vi "Motion Status Reader.vi"(8 "error in (no error)":errorcluster, 11 "Control":refnum<notifier>) -> ()   [LabVIEW 2015, in "Tool Module.lvlib"]
uses:
  Tool Module.lvlib
  Tool Interface/_Host - HS Data Stream State Enum Typedef.ctl
  _Motion Status Reader SM enum--typedef.ctl
  Tool Typedefs/_Motion STATUS Cluster--typedef.ctl
  Tool Interface/GLOB - Configuration Options.vi
  Support/ToolModGLOB.vi
  Tool Interface/Tool Interface.lvlib
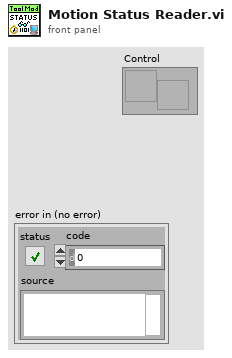
[diagram p1: front panel]
types:
  T1 = typedef "Tool Module.lvlib/_Motion Status Reader SM enum--typedef.ctl" = enum16{"Not Connected", "Connect", "Idle", "Receive Data", "Disconnect"}
  T2 = typedef "Tool Interface.lvlib/_Host - HS Data Stream State Enum Typedef.ctl" = enum16{"Idle", "Connect", "Receive Data", "Close Connection"}
  T3 = typedef "_Motion STATUS Cluster--typedef.ctl" = cluster{"Encoder":i32, "STATUS":u16, "MC SM State":u16, "M_Ctrl":u16}
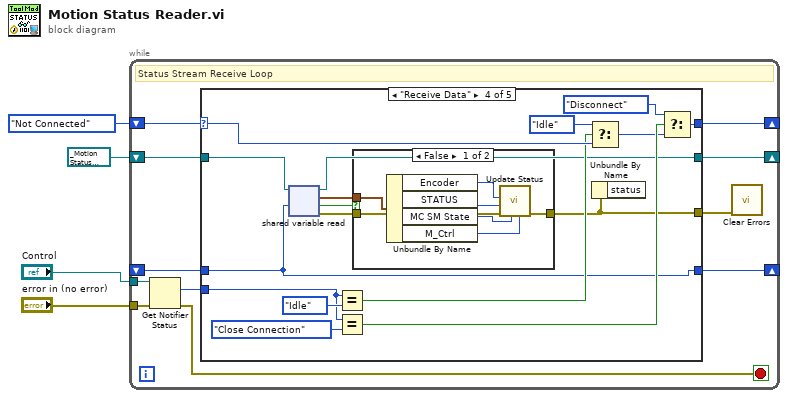
[diagram p0: block diagram]
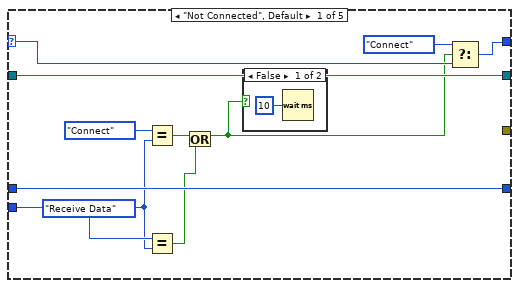
[diagram p2: hidden frame]
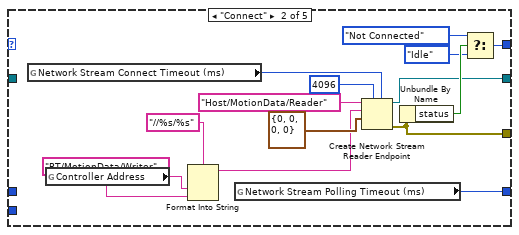
[diagram p4: hidden frame]
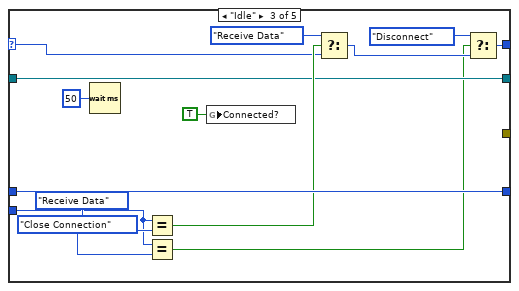
[diagram p5: hidden frame]
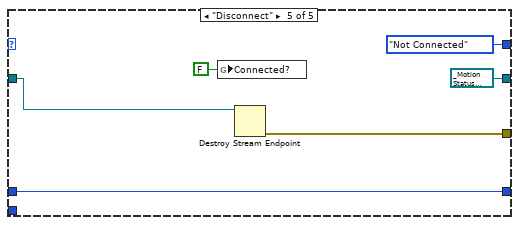
[diagram p7: hidden frame]
diagram:
  n1 = while {
    shift-right: [w14] -> _
    shift-left: _ -> [w13]
    shift-right: [w12] -> _
    shift-left: refnum<k21> refnum ("reader endpoint") -> [w7]
    tunnel: "Control" -> [w11]
    shift-right: [w9] -> _
    shift-left: _Motion_Status_Reader_SM_enum--typedef."Not Connected" ("_Motion Status Reader SM Enum--typedef") -> [w15]
    tunnel: "error in (no error)" -> [w6]
    stop <- w5 stop-if-true
    # "Status Stream Receive Loop"
    n2 = Get Notifier Status(notifier=w11, error in (no error)=w6) -> (current notification=w10:T2, error out=w5:errorcluster)  [unwired: 3 out]
    n3 = case shown="\"Receive Data\"" w15 {
      selector: w15 -> [w26 _ w53 w72 _]
      tunnel: [w23 w34 w55 w61 w84] -> w14
      tunnel: w13 -> [w23 _ w55 w61 w84]
      tunnel: [w22 w28 w51 w62 refnum<k21> refnum ("reader endpoint")] -> w12
      tunnel: w10 -> [w18 _ w44 w68 _]
      tunnel: [w25 w32 w50 w70 _Motion_Status_Reader_SM_enum--typedef."Not Connected" ("_Motion Status Reader SM Enum--typedef")] -> w9
      tunnel: [_ w33 _ w57 w85] -> w8
      tunnel: w7 -> [w22 _ w51 w63 w87]
      frame "Not Connected", Default {
        n4 = Equal?(x=_Host_-_HS_Data_Stream_State_Enum_Typedef."Connect", y=w18) -> (x = y?=w20:bool)
        n5 = Equal?(x=_Host_-_HS_Data_Stream_State_Enum_Typedef."Receive Data", y=w18) -> (x = y?=w16:bool)
        n6 = Or(x=w20, y=w16) -> (x .or. y?=w17:bool)
        n7 = case shown="False" w17 {
          frame False {
            n8 = Wait (ms)(milliseconds to wait=u32 10) -> ()  [unwired: 1 out]
          }
          frame True {
          }
        }
        n9 = Select(t=_Motion_Status_Reader_SM_enum--typedef."Connect", s=w17, f=w26) -> (s? t:f=w25:T1)
      }
      frame "Connect" {
        n10 = global read "GLOB - Configuration Options.vi" "Network Stream Connect Timeout (ms)"() -> (w39:i32)
        n11 = global read "GLOB - Configuration Options.vi" "Controller Address"() -> (w42:string)
        n12 = Format Into String(format string="//%s/%s", w42, "RT/MotionData/Writer" ("input 2")) -> (resulting string=w38:string)  [unwired: 2 in, 1 out]
        n13 = global read "GLOB - Configuration Options.vi" "Network Stream Polling Timeout (ms)"() -> (w34:i32)
        n14 = Create Network Stream Reader Endpoint(5:w39, 7:4096 ("reader buffer size"), 9:T3 {"Encoder"=0, "STATUS"=0, "MC SM State"=0, "M_Ctrl"=0} ("_Motion Status Cluster--typedef"), 10:w38, 11:"Host/MotionData/Reader" ("reader name")) -> (0:w33:errorcluster, 3:w28:refnum<k21>)  [unwired: 2 in]
        n15 = Unbundle By Name(w33) -> ("status"=w31:bool)
        n16 = Select(t=_Motion_Status_Reader_SM_enum--typedef."Not Connected", s=w31, f=_Motion_Status_Reader_SM_enum--typedef."Idle") -> (s? t:f=w32:T1)
      }
      frame "Idle" {
        n17 = Wait (ms)(milliseconds to wait=u32 50) -> ()  [unwired: 1 out]
        n18 = Equal?(x=w44, y=_Host_-_HS_Data_Stream_State_Enum_Typedef."Receive Data" ("x")) -> (x = y?=w54:bool)
        n19 = Equal?(x=w44, y=_Host_-_HS_Data_Stream_State_Enum_Typedef."Close Connection" ("x")) -> (x = y?=w47:bool)
        n20 = global write "ToolModGLOB.vi" "Connected?"(TRUE ("Connected?")) -> ()
        n21 = Select(t=_Motion_Status_Reader_SM_enum--typedef."Receive Data", s=w54, f=w53) -> (s? t:f=w49:T1)
        n22 = Select(t=_Motion_Status_Reader_SM_enum--typedef."Disconnect", s=w47, f=w49) -> (s? t:f=w50:T1)
      }
      frame "Receive Data" {
        n23 = shared-variable-read(w63, w61) -> (w62:refnum<k21>, w60:errorcluster, w58:bool, w59:T3)  [unwired: 1 in]
        n24 = Equal?(x=w68, y=_Host_-_HS_Data_Stream_State_Enum_Typedef."Idle" ("x")) -> (x = y?=w69:bool)
        n25 = Equal?(x=w68, y=_Host_-_HS_Data_Stream_State_Enum_Typedef."Close Connection") -> (x = y?=w66:bool)
        n26 = case shown="False" w58 {
          tunnel: w60 -> [w80 w81]
          tunnel: [w76 w81] -> w57
          tunnel: w59 -> [w79 _]
          frame False {
            n27 = Unbundle By Name(w79) -> ("Encoder"=w78:i32, "STATUS"=w77:u16, "MC SM State"=w75:u16, "M_Ctrl"=w74:u16)
            n28 = call "Update Status.vi"("M_Ctrl"=w74, "MC SM State"=w75, "error in (no error)"=w80, "STATUS"=w77, "Encoder"=w78) -> ("error out"=w76:errorcluster)  [unwired: 6 in]
          }
          frame True {
          }
        }
        n29 = Select(t=_Motion_Status_Reader_SM_enum--typedef."Idle", s=w69, f=w72) -> (s? t:f=w65:T1)
        n30 = Unbundle By Name(w57) -> ()  [unwired: 1 out]
        n31 = Select(t=_Motion_Status_Reader_SM_enum--typedef."Disconnect", s=w66, f=w65) -> (s? t:f=w70:T1)
      }
      frame "Disconnect" {
        n32 = global write "ToolModGLOB.vi" "Connected?"(FALSE ("Connected?")) -> ()
        n33 = Destroy Stream Endpoint(11:w87) -> (0:w85:errorcluster)  [unwired: 1 in]
      }
    }
    n34 = call <vilib>:"Clear Errors.vi"("error in (no error)"=w8) -> ()  [unwired: 5 in, 2 out]
  }
